vi "protocol.vi"(10 "数值":i32 format="%x") -> (2 "字符串":string)   [LabVIEW 2018]
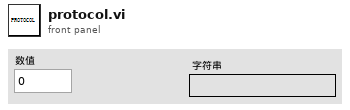
[diagram p1: front panel]
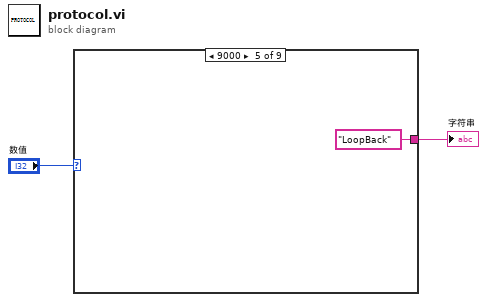
[diagram p0: block diagram]
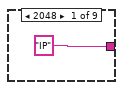
[diagram p2: hidden frame]
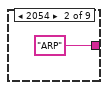
[diagram p3: hidden frame]
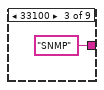
[diagram p4: hidden frame]
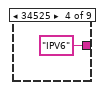
[diagram p5: hidden frame]
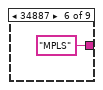
[diagram p6: hidden frame]
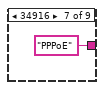
[diagram p7: hidden frame]
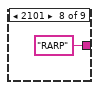
[diagram p8: hidden frame]
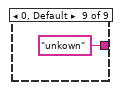
[diagram p9: hidden frame]
diagram:
  n1 = case shown="9000" "数值" {
    tunnel: ["IP" "ARP" "SNMP" "IPV6" "LoopBack" "MPLS" "PPPoE" "RARP" "unkown"] -> w1
    frame 2048 {
    }
    frame 2054 {
    }
    frame 33100 {
    }
    frame 34525 {
    }
    frame 36864 {
    }
    frame 34887 {
    }
    frame 34916 {
    }
    frame 2101 {
    }
    frame 0, Default {
    }
  }
  "字符串" <- w1
